vi "PH_Sixpack.Action Operation.vi"(0 "VI in":refnum<vi>, 5 "error in":errorcluster) -> (14 "VI out":refnum<vi>, 19 "error out":errorcluster)   [LabVIEW 2014, in "PH_Sixpack.lvlib"]
doc: "This VI is made to act on 6P hardware in a certain state. It is used in ProcPrdc."
uses:
  PH_Sixpack.lvlib
  PH_Basics/PH_Stepmotor_BaseClass/PH_Stepmotor_BaseClass.lvlib
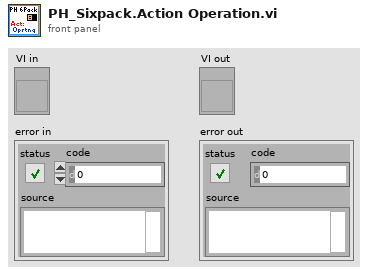
[diagram p1: front panel]
types:
  T1 = typedef "PH_Sixpack.lvlib/PH_Sixpack.Status.ctl" = enum32{"None", "Init", "Configure", "configured", "Close", "closed"}
  T2 = typedef "PH_Stepmotor_BaseClass.lvlib/PH_Stepmotor_BaseClass.i attribute.ctl" = cluster{"Device Error":errorcluster, "Axes PSDB Thread":cluster{"Ref":refnum<vi>, "Q-Ref":refnum<queue>, "Data Status":T3}, "Axes":T4[], "Axes PSDB Infos":cluster{"GUI Name":string, "PSDB Instance ID":i32, "PSDB Status Service ID":i32, "Axis":i32, "Class":string}[], "GUI Refs":T9}
  T3 = typedef "PH_PSDBWriter.lvlib/PH_PSDBWriter.Data Status.ctl" = i16
  T4 = typedef "PH_Stepmotor_BaseClass.lvlib/PH_Stepmotor_BaseClass.Axis Attributes.ctl" = cluster{"Settings":T5, "Endswitch?":bool, "DIM Service IDs":T7, "Activity":T8, "Configured?":bool, "Position":cluster{"Current":i32, "Target":i32}, "Position to set":cluster{"New?":bool, "Wanted":i32}, "Stop?":bool, "Reset?":bool, "Move?":bool, "Nothing connected?":bool}
  T5 = typedef "PH_Stepmotor_BaseClass.lvlib/PH_Stepmotor_BaseClass.Axis Settings.ctl" = cluster{"Sign change":bool, "Width":dbl, "Calibration":dbl, "Unit":string, "Motor Type":T6, "Unit Width":string, "Unit CF":string}
  T6 = typedef "PH_Stepmotor_BaseClass.lvlib/PH_Stepmotor_BaseClass.Motor Type.ctl" = enum16{"Unspecific", "OWIS 49.120.2633", "OWIS 49.060.1033", "OWIS 43.040.2558", "Diamond Motion 2200 series", "OWIS 49.120.266B.MV6", "Calorimeter", "Linear Stage 1", "MICOS VT-80", "MICOS VT-80 S", "Standa Rotstage nt0.95A", "PUF RA 320.200", "PUF RA 800.200", "PUF RA 800.400", "PUF RA 400.50", "1324.nn.800.50", "1324.n9c.800.50", "1324.nn.320.200", "1324.nn.400.200", "1324.nn.800.200", "1324.nn.400.50", "1324.8c9c.800.50", "1324.8c9c.400.200"}
  T7 = typedef "PH_Stepmotor_BaseClass.lvlib/PH_Stepmotor_BaseClass.Axis DIM Service IDs.ctl" = cluster{"Settings":i32, "Information":i32}
  T8 = typedef "PH_Stepmotor_BaseClass.lvlib/PH_Stepmotor_BaseClass.Axis Activity.ctl" = enum16{"No Information", "stopped", "running", "Failure", "Alarm", "stopped at backward ES", "stopped at foreward ES"}
  T9 = typedef "PH_Stepmotor_BaseClass.lvlib/PH_Stepmotor_BaseClass.GUI Refs.ctl" = cluster{"Axes Configuration":refnum<vi>, "Device Error":refnum<vi>, "Axes PSDB Infos":refnum<vi>}
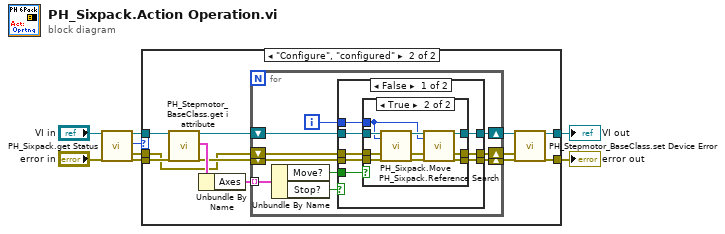
[diagram p0: block diagram]
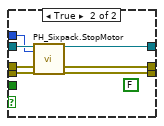
[diagram p4: hidden frame]
diagram:
  n1 = call "PH_Sixpack.get Status.vi"("VI in"="VI in", "error in (no error)"="error in") -> ("VI out"=w5:refnum<vi>, "Status"=w2:T1, "Device Error"=w1:errorcluster, "error out"=w3:errorcluster)  [unwired: 14 in]
  n2 = case shown="\"Configure\", \"configured\"" w2 {
    tunnel: w5 -> [w10 w17]
    tunnel: w3 -> [w9 w22]
    tunnel: [w9 w11] -> w8
    tunnel: [w10 w12] -> w7
    tunnel: w1 -> [_ w16]
    frame Default {
    }
    frame "Configure", "configured" {
      n3 = call "PH_Stepmotor_BaseClass.get i attribute.vi"("i ref in"=w17, "error in (no error)"=w22) -> ("i ref out"=w19:refnum<vi>, "i attribute"=w21:T2, "error out"=w18:errorcluster)  [unwired: 15 in]
      n4 = Unbundle By Name(w21) -> ("Axes"=w20:T4[])
      n5 = for {
        tunnel: w20 -> [w32] mode=indexing
        shift-right: [w26] -> w13
        shift-left: w19 -> [w31]
        shift-right: [w24] -> w15
        shift-left: w18 -> [w30]
        shift-right: [w25] -> w14
        shift-left: w16 -> [w29]
        i -> [w27]
        n6 = Unbundle By Name(w32) -> ("Move?"=w23:bool, "Stop?"=w28:bool)
        n7 = case shown="False" w28 {
          tunnel: w31 -> [w40 w60]
          tunnel: [w39 w59] -> w26
          tunnel: w30 -> [w37 w58]
          tunnel: [w35 w57] -> w24
          tunnel: w29 -> [w38 w56]
          tunnel: [w36 w55] -> w25
          tunnel: w27 -> [w34 w54]
          tunnel: w23 -> [w33 _]
          frame False {
            n8 = case shown="True" w33 {
              tunnel: w40 -> [w43 w52]
              tunnel: w38 -> [w42 w53]
              tunnel: w37 -> [w41 w51]
              tunnel: [w43 w45] -> w39
              tunnel: [w41 w47] -> w35
              tunnel: [w42 w49] -> w36
              tunnel: w34 -> [_ w44]
              frame False {
              }
              frame True {
                n9 = call "PH_Sixpack.Move.vi"("i ref in"=w52, "axis"=w44, "Device Error in"=w53, "error in"=w51) -> ("i ref out"=w46:refnum<vi>, "Device Error out"=w50:errorcluster, "error out"=w48:errorcluster)  [unwired: 13 in]
                n10 = call "PH_Sixpack.Reference Search.vi"("i ref in"=w46, "axis"=w44, "Device Error in"=w50, "error in"=w48) -> ("i ref out"=w45:refnum<vi>, "Device Error out"=w49:errorcluster, "error out"=w47:errorcluster)  [unwired: 13 in]
              }
            }
          }
          frame True {
            (unwired) FALSE
            n11 = call "PH_Sixpack.StopMotor.vi"("i ref in"=w60, "axis"=w54, "Device Error in"=w56, "error in"=w58) -> ("i ref out"=w59:refnum<vi>, "Device Error out"=w55:errorcluster, "error out"=w57:errorcluster)  [unwired: 13 in]
          }
        }
      }
      n12 = call "PH_Stepmotor_BaseClass.set Device Error.vi"("i ref in"=w13, "Device Error"=w14, "error in"=w15) -> ("i ref out"=w12:refnum<vi>, "error out"=w11:errorcluster)  [unwired: 15 in]
    }
  }
  "error out" <- w8
  "VI out" <- w7
